vi "AutonomousScript.vi"() -> ()   [LabVIEW 2015]
panel:
  out "current command":string
  out "GrabValue":dbl
  out "Z":u8(slide) scale=0.0..100.0
  out "Y":dbl(slide) scale=0.0..1.0
  out "X":dbl(slide) scale=0.0..1.0
  out "Script":string="drive .3 .4 .0\nwait 2000\nstop\nwait 3000\ndrive .1 .2 .3\nwait 5000\nstop\nwait 1000\nlift .75\nwait 3600\nstop\n\n"
  out "LiftValue":dbl
  out "Wait Time":i32
  out "Z":dbl
  out "Y":dbl
  out "X":dbl
  out "Mode":string
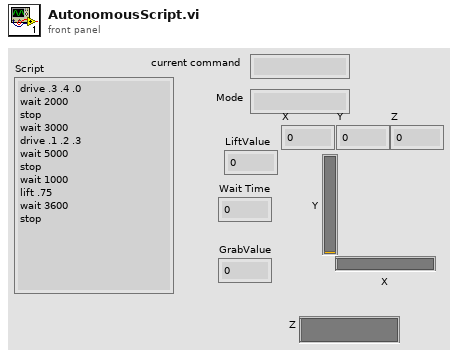
[diagram p1: front panel]
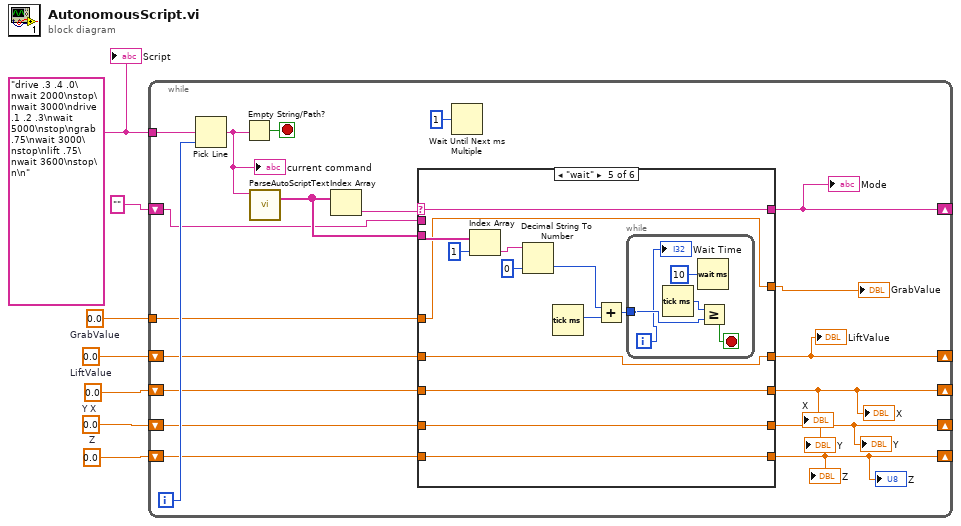
[diagram p0: block diagram]
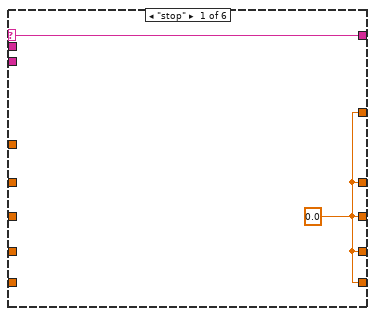
[diagram p2: hidden frame]
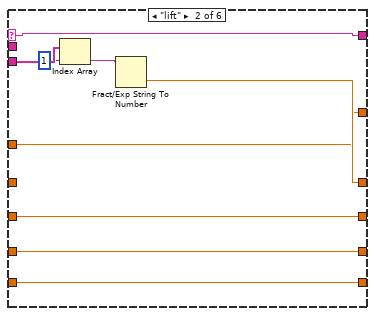
[diagram p3: hidden frame]
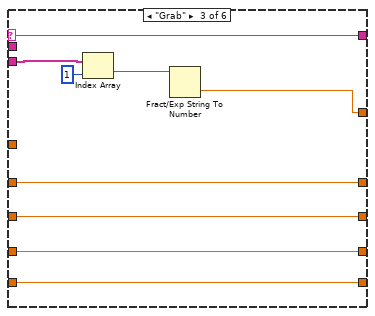
[diagram p4: hidden frame]
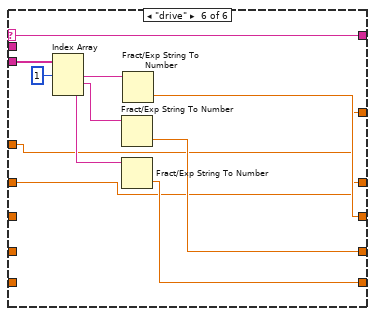
[diagram p6: hidden frame]
diagram:
  w1 = 0.0  # GrabValue
  w2 = 0.0  # LiftValue
  w4 = 0.0  # Z
  w5 = 0.0  # Y
  w6 = 0.0  # X
  w7 = "drive .3 .4 .0\nwait 2000\nstop\nwait 3000\ndrive .1 .2 .3\nwait 5000\nstop\ngrab .75\nwait 3000\nstop\nlift .75\nwait 3600\nstop\n\n"
  n1 = while {
    tunnel: w7 -> [w25]
    shift-right: [w13] -> _
    shift-left: w6 -> [w20]
    shift-right: [w12] -> _
    shift-left: w5 -> [w19]
    shift-right: [w11] -> _
    shift-left: w4 -> [w18]
    shift-right: [w16] -> _
    shift-left: "" -> [w17]
    shift-right: [w14] -> _
    shift-left: w2 -> [w15]
    tunnel: w1 -> [w9]
    i -> [w26]
    stop <- w24 stop-if-true
    n2 = Pick Line(multi-line string=w25, line index=w26) -> (output string=w23:string)  [unwired: 1 in]
    "current command" <- w23
    n3 = Empty String/Path?(string/path=w23) -> (empty?=w24:bool)
    n4 = call "ParseAutoScriptText.vi"("output string"=w23) -> ("Array"=w21:string[])  [unwired: 10 in]
    n5 = Index Array(array=w21) -> (element=w22:string)  [unwired: 1 in]
    n6 = case shown="\"wait\"" w22 {
      selector: w22 -> [w28 w32 w44 _ w55 w73]
      tunnel: w21 -> [_ w34 w45 _ w65 w81]
      tunnel: w20 -> [_ w37 w42 w51 w58 _]
      tunnel: [w27 w37 w42 w51 w58 w76] -> w13
      tunnel: w19 -> [_ w36 w41 w50 w57 _]
      tunnel: [w27 w36 w41 w50 w57 w75] -> w12
      tunnel: w18 -> [_ w35 w40 w49 w56 _]
      tunnel: [w27 w35 w40 w49 w56 w74] -> w11
      tunnel: w17 -> [_ _ _ w52 _ _]
      tunnel: [w28 w32 w44 w52 w55 w73] -> w16
      tunnel: w15 -> [_ _ w43 w48 w54 w72]
      tunnel: [w27 w30 w43 w48 w54 w72] -> w14
      tunnel: [w27 w29 w38 w47 w53 w71] -> w10
      tunnel: w9 -> [_ w29 _ w47 w53 w71]
      frame "stop" {
        w27 = 0.0 ("X")
      }
      frame "lift" {
        n7 = Index Array(array=w34, index=1) -> (element=w31:string)
        n8 = Fract/Exp String To Number(string=w31) -> (number=w30:dbl)  [unwired: 3 in, 1 out]
      }
      frame "Grab" {
        n9 = Index Array(array=w45, index=1) -> (element=w39:string)
        n10 = Fract/Exp String To Number(string=w39) -> (number=w38:dbl)  [unwired: 3 in, 1 out]
      }
      frame "null", Default {
      }
      frame "wait" {
        n11 = Index Array(array=w65, index=1) -> (element=w63:string)
        n12 = Decimal String To Number(string=w63, default (0L)=u32 0 ("default (0 I32)")) -> (number=w61:u32)  [unwired: 1 in, 1 out]
        n13 = Tick Count (ms)() -> (millisecond timer value=w62:u32)
        n14 = Add(x=w61, y=w62) -> (x+y=w60:u32)
        n15 = while {
          tunnel: w60 -> [w67]
          i -> [w66]
          stop <- w69 stop-if-true
          n16 = Tick Count (ms)() -> (millisecond timer value=w68:u32)
          n17 = Wait (ms)(milliseconds to wait=u32 10) -> ()  [unwired: 1 out]
          n18 = Greater Or Equal?(x=w68, y=w67) -> (x >= y?=w69:bool)
          "Wait Time" <- w66
        }
      }
      frame "drive" {
        n19 = Index Array(array=w81, index #1=1 ("index")) -> (element #1=w79:string, element #2=w78:string, element #3=w77:string)  [unwired: 2 in]
        n20 = Fract/Exp String To Number(string=w78) -> (number=w75:dbl)  [unwired: 3 in, 1 out]
        n21 = Fract/Exp String To Number(string=w77) -> (number=w74:dbl)  [unwired: 3 in, 1 out]
        n22 = Fract/Exp String To Number(string=w79) -> (number=w76:dbl)  [unwired: 3 in, 1 out]
      }
    }
    "X" <- w13
    "Y" <- w12
    "Z" <- w11
    "Mode" <- w16
    "LiftValue" <- w14
    "X" <- w13
    "Y" <- w12
    "Z" <- w11
    "GrabValue" <- w10
    n23 = Wait Until Next ms Multiple(millisecond multiple=u32 1) -> ()  [unwired: 1 out]
  }
  "Script" <- w7
